vi "Create Bucket.vi"(6 "Access Control List":T1, 8 "error in (no error)":errorcluster, 9 "Region":T2, 10 "Name":string, 11 "AWS Credentials":T3) -> (0 "error out":errorcluster, 3 "Bucket out":refnum<class "Bucket.lvclass">)   [LabVIEW 2015, in "NI_AWS_S3.lvlib" / "Bucket.lvclass"]
uses:
  Bucket.lvclass
  Core/HTTP Request/AWS Credentials.ctl
  Core/HTTP Request/Region.ctl
  ACL.ctl
  Core/HTTP Request/Request Options.ctl
  Core/HTTP Request/Name Value Pair.ctl
  Core/HTTP Request/Region handling.ctl
  Core/HTTP Request/URL formatting.ctl
  Core/HTTP Request/HTTP Request.lvclass/HTTP Request.ctl
  Bucket.lvclass/Bucket.ctl
  Core/HTTP Request/Write Credentials.vi
  Core/HTTP Request/Write Region.vi
  Core/HTTP Request/Write Service.vi
  Core/HTTP Request/Write Verify Server.vi
  Write Name.vi
  Core/HTTP Request/HTTP Request.lvclass
  NI_AWS_S3.lvlib
panel:
  out "Body":string
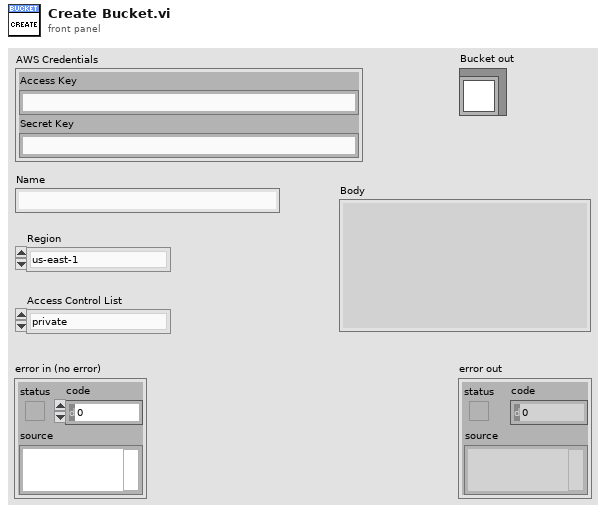
[diagram p1: front panel]
types:
  T1 = typedef "NI_AWS_S3.lvlib/ACL.ctl" = enum16{"private", "public-read", "public-read-write", "aws-exec-read", "authenticated-read", "bucket-owner-read", "bucket-owner-full-control"}
  T2 = typedef "NI_AWS_Core.lvlib/HTTP Request.lvclass/Region.ctl" = enum16{"us-east-1", "us-east-2", "us-west-1", "us-west-2", "ap-northeast-1", "ap-northeast-2", "ap-southeast-1", "ap-southeast-2", "ca-central-1", "eu-central-1", "eu-west-1", "eu-west-2", "sa-east-1"}
  T3 = typedef "NI_AWS_Core.lvlib/HTTP Request.lvclass/AWS Credentials.ctl" = cluster{"Access Key":string, "Secret Key":string}
  T4 = typedef "NI_AWS_Core.lvlib/HTTP Request.lvclass/Region handling.ctl" = enum16{"use region everywhere", "use region (authentication only)", "use region (URL only)", "ignore region everwhere"}
  T5 = typedef "NI_AWS_Core.lvlib/HTTP Request.lvclass/Request Options.ctl" = cluster{"request headers":T6[], "request parameters":T6[], "request body":string, "region handling":T4, "URL formatting":T7}
  T6 = typedef "NI_AWS_Core.lvlib/HTTP Request.lvclass/Name Value Pair.ctl" = cluster{"name":string, "value":string}
  T7 = typedef "NI_AWS_Core.lvlib/HTTP Request.lvclass/URL formatting.ctl" = enum16{"region-", "region."}
  T8 = typedef "NI_AWS_Core.lvlib/HTTP Request.lvclass/Response.ctl" = cluster{"Headers":string, "Body":string}
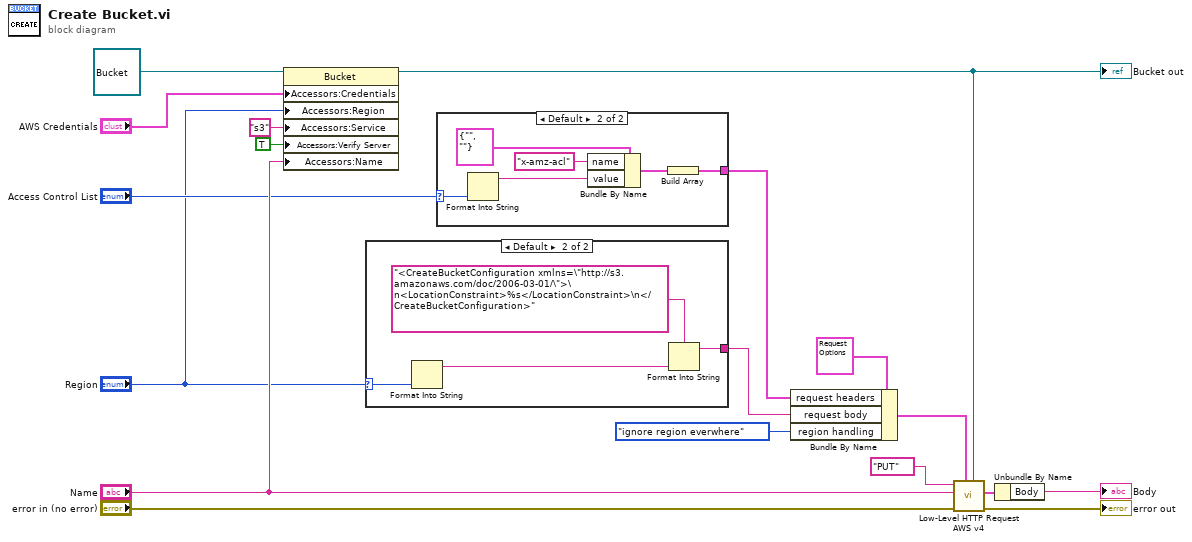
[diagram p0: block diagram]
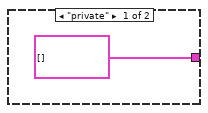
[diagram p3: hidden frame]
diagram:
  n1 = property class="Bucket"(reference=refnum<class "Bucket.lvclass"> refnum ("NI_AWS_S3.lvlib:Bucket.lvclass"), "Accessors:Credentials"="AWS Credentials", "Accessors:Region"="Region", "Accessors:Service"="s3" ("Service"), "Accessors:Verify Server"=TRUE ("Verify Server"), "Accessors:Name"="Name") -> (reference out=w11:refnum<class "Bucket.lvclass">)  [unwired: 1 in, 1 out]
  "Bucket out" <- w11
  n2 = case shown="Default" "Region" {
    selector: "Region" -> [_ w22]
    tunnel: [_ w19] -> w1
    frame "us-east-1" {
    }
    frame Default {
      n3 = Format Into String(w22) -> (resulting string=w20:string)  [unwired: 3 in, 1 out]
      n4 = Format Into String(format string="<CreateBucketConfiguration xmlns=\"http://s3.amazonaws.com/doc/2006-03-01/\">\n<LocationConstraint>%s</LocationConstraint>\n</CreateBucketConfiguration>", w20) -> (resulting string=w19:string)  [unwired: 2 in, 1 out]
    }
  }
  n5 = case shown="Default" "Access Control List" {
    selector: "Access Control List" -> [_ w25]
    tunnel: [T6[] [] w26] -> w3
    frame "private" {
    }
    frame Default {
      n6 = Format Into String(w25) -> (resulting string=w24:string)  [unwired: 3 in, 1 out]
      n7 = Bundle By Name(cluster=T6 {"name"="", "value"=""} ("Name Value Pair"), "name"="x-amz-acl" ("Header"), "value"=w24) -> (w27:T6)
      n8 = Build Array(w27) -> (w26:T6[])
    }
  }
  n9 = Bundle By Name(cluster=T5 {"request headers"=[], "request parameters"=[], "request body"="", "region handling"=enum."use region everywhere", "URL formatting"=enum."region."} ("Request Options"), "request headers"=w3, "request body"=w1, "region handling"=Region_handling."ignore region everwhere") -> (w8:T5)
  n10 = call "Low-Level HTTP Request AWS v4.vi"("AWS Core"=w11, "Request Options"=w8, "error in (no error)"="error in (no error)", "URL Prefix"="Name", "HTTP-Verb"="PUT") -> ("error out"=→"error out":errorcluster, "Response"=w18:T8)  [unwired: 4 in, 1 out]
  n11 = Unbundle By Name(w18) -> ("Body"=→"Body":string)
